vi "Test B.vi"(8 "error in (no error)":errorcluster) -> (0 "error out":errorcluster)   [LabVIEW 2019, in "Simple Example(Station2).lvlib"]
uses:
  400e6fd7-5c57-4563-98c8-4c487ac03ebd.vi
  d135eecd-02d8-4d26-94c7-1196041114e8.vi
  LVUT Global 1.vi
  <vilib>/Utility/Data Type/Get Type Information.vi
  <vilib>/Utility/error.llb/Trim Whitespace.vi
  Almost Equal.vi
  Simple Example(Station2).lvlib
  Unit Test Engine Tools.lvlib
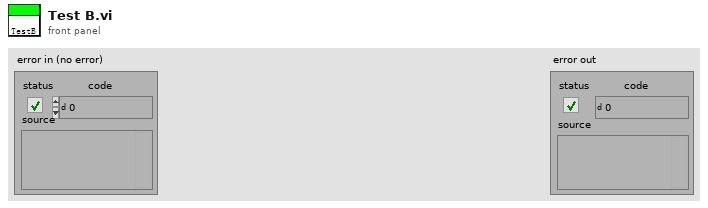
[diagram p1: front panel]
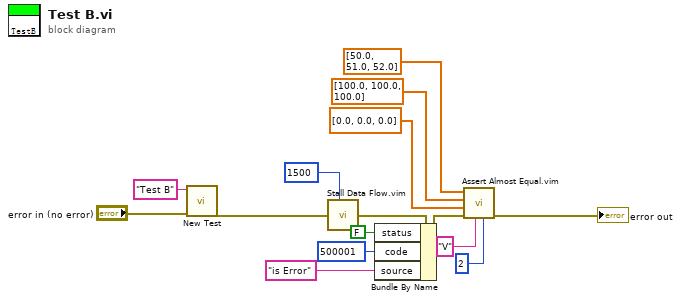
[diagram p0: block diagram]
diagram:
  n1 = call "New Test.vi"("error in (no error)"="error in (no error)", "Test"="Test B") -> ("error out"=w13:errorcluster)  [unwired: 9 in]
  n2 = call "Stall Data Flow.vim"("value in"=w13, "milliseconds to wait"=u32 1500) -> ("value out"=w10:errorcluster)  [unwired: 1 out]
  n3 = Bundle By Name(cluster=w10, "status"=FALSE, "code"=500001, "source"="is Error") -> (w5:errorcluster)
  n4 = call "Assert Almost Equal.vim"("precision (2)"=i16 2 ("precision (6)"), "Unit"="V", "error in (no error)"=w5, "a"=dbl[] [0.0, 0.0, 0.0], "b"=dbl[] [100.0, 100.0, 100.0], "x"=dbl[] [50.0, 51.0, 52.0]) -> ("error out"=→"error out":errorcluster)  [unwired: 5 in]
